vi "Request Display Charm.vi"(8 "error in (no error)":errorcluster, 11 "Sensor in":refnum<class "Sensor.lvclass">) -> (0 "error out":errorcluster, 3 "Sensor out":refnum<class "Sensor.lvclass">)   [LabVIEW 2012, in "Sensor Definition.lvlib" / "Sensor.lvclass"]
uses:
  Sensor.lvclass
  Win8uiFramework/Display Charm Msg.lvclass
  <vilib>/ActorFramework/Actor/Actor.lvclass
  SensorCharm.lvclass
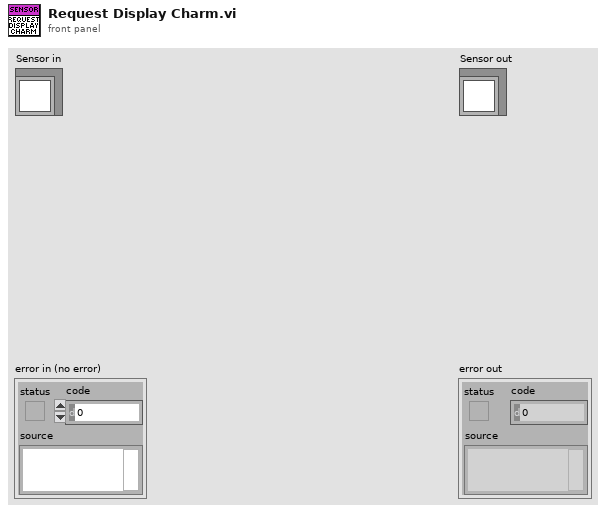
[diagram p1: front panel]
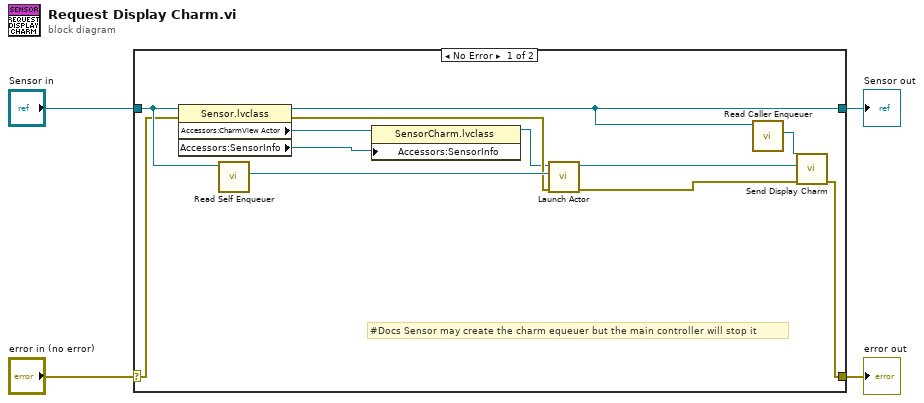
[diagram p0: block diagram]
diagram:
  n1 = case shown="No Error" "error in (no error)" {
    selector: "error in (no error)" -> [w9 w18]
    tunnel: [w10 w18] -> w3
    tunnel: [w16 w17] -> w1
    tunnel: "Sensor in" -> [w15 w17]
    frame No Error {
      # "#Docs Sensor may create the charm equeuer but the main controller will stop it"
      n2 = property class="Sensor.lvclass"(reference=w15, error in=w9) -> (reference out=w16:refnum<class "Sensor.lvclass">, error out=w13:errorcluster, "Accessors:CharmView Actor"=w6:refnum<class "SensorCharm.lvclass">, "Accessors:SensorInfo"=w5:refnum<class "SensorInfo.lvclass">)
      n3 = call <vilib>:"Read Self Enqueuer.vi"("Actor"=w15) -> ("Self Enqueuer"=w14:refnum<class "Message Enqueuer.lvclass">)  [unwired: 10 in]
      n4 = property class="SensorCharm.lvclass"(reference=w6, "Accessors:SensorInfo"=w5) -> (reference out=w7:refnum<class "SensorCharm.lvclass">)  [unwired: 1 in, 1 out]
      n5 = call <vilib>:"Launch Actor.vi"("error in (no error)"=w13, "Actor-to-Caller Enqueuer"=w14, "Actor"=w7) -> ("error out"=w8:errorcluster, "Caller-To-Actor Enqueuer"=w12:refnum<class "Message Enqueuer.lvclass">)  [unwired: 7 in]
      n6 = call <vilib>:"Read Caller Enqueuer.vi"("Actor"=w16) -> ("Caller Enqueuer"=w11:refnum<class "Message Enqueuer.lvclass">)  [unwired: 10 in]
      n7 = call "Send Display Charm.vi"("error in (no error)"=w8, "Charm Enqueuer"=w12, "Message Enqueuer"=w11) -> ("error out"=w10:errorcluster)  [unwired: 7 in, 1 out]
    }
    frame Error {
    }
  }
  "error out" <- w3
  "Sensor out" <- w1
